vi "Configure Time Slot.vi"(6 "Exclusion Duration Interval (0 s)":dbl, 7 "Slot Duration (0.0001 s)":dbl=0.0001, 8 "error in (no error)":errorcluster, 9 "End Time (0 %)":dbl, 10 "Start Time (0 %)":dbl, 11 "VISA resource name":refnum<visa-resource-name>) -> (0 "error out":errorcluster, 3 "VISA resource name out":refnum<visa-resource-name>)   [LabVIEW 2014, in "Agilent U2000 Series.lvlib"]
doc: "Sets the slot duration, the measurement gate start and end time and the exclusion duration interval within the time slot. \n\nNote: \nThis VI is only applicable for U2042XA/U2044XA/U2049XA."
uses:
  Agilent U2000 Series.lvlib
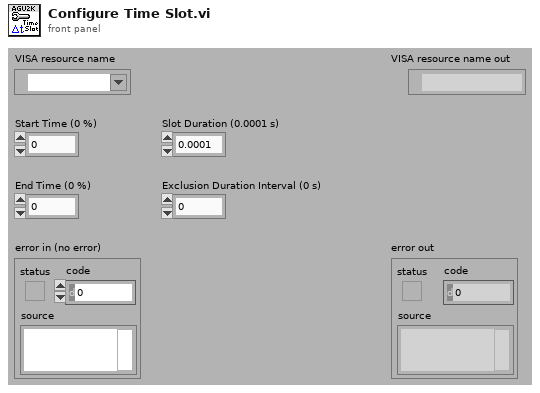
[diagram p1: front panel]
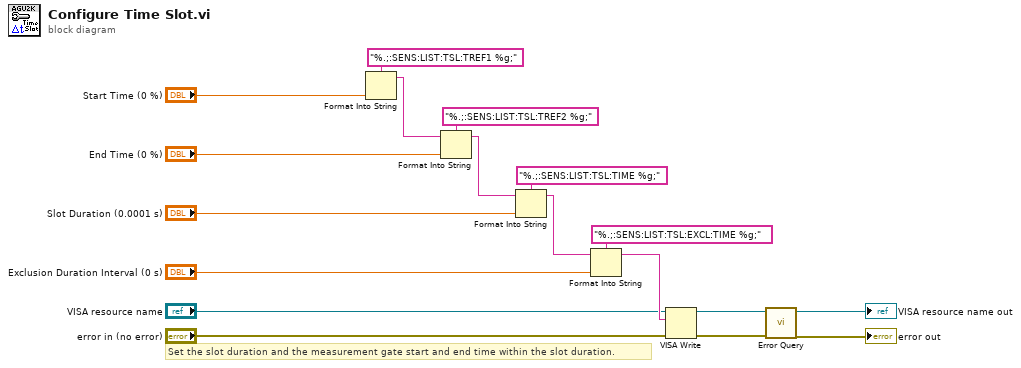
[diagram p0: block diagram]
diagram:
  # "Set the slot duration and the measurement gate start and end time within the slot duration."
  n1 = Format Into String(format string="%.;:SENS:LIST:TSL:TREF1 %g;", "Start Time (0 %)") -> (resulting string=w16:string)  [unwired: 2 in, 1 out]
  n2 = Format Into String(format string="%.;:SENS:LIST:TSL:TREF2 %g;", initial string=w16, "End Time (0 %)") -> (resulting string=w13:string)  [unwired: 1 in, 1 out]
  n3 = Format Into String(format string="%.;:SENS:LIST:TSL:TIME %g;", initial string=w13, "Slot Duration (0.0001 s)") -> (resulting string=w10:string)  [unwired: 1 in, 1 out]
  n4 = Format Into String(format string="%.;:SENS:LIST:TSL:EXCL:TIME %g;", initial string=w10, "Exclusion Duration Interval (0 s)") -> (resulting string=w7:string)  [unwired: 1 in, 1 out]
  n5 = VISA Write(VISA resource name="VISA resource name", write buffer=w7, error in (no error)="error in (no error)") -> (VISA resource name out=w4:refnum<visa-resource-name>, error out=w3:errorcluster)  [unwired: 1 out]
  n6 = call "Error Query.vi"("error in (no error)"=w3, "VISA resource name"=w4) -> ("error out"=→"error out":errorcluster, "VISA resource name out"=→"VISA resource name out":refnum<visa-resource-name>)  [unwired: 6 in, 2 out]
